vi "Settings.vi"(9 "Debug":bool, 10 "AeroQuad Flight Software Folder":path, 11 "Arduino IDE Folder":path) -> (1 "Debug Out":bool, 2 "Flight Software Path":path, 3 "IDE Path":path)   [LabVIEW 2010]
panel:
  in  "Cancel":bool
  in  "OK":bool
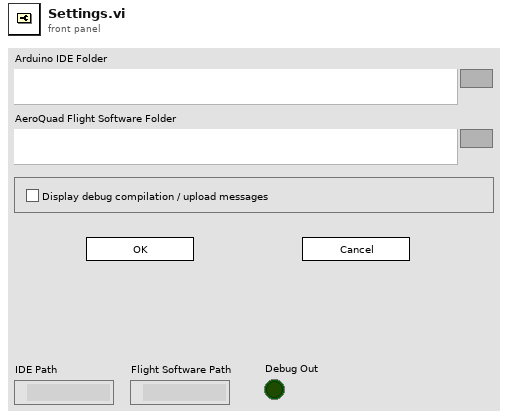
[diagram p1: front panel]
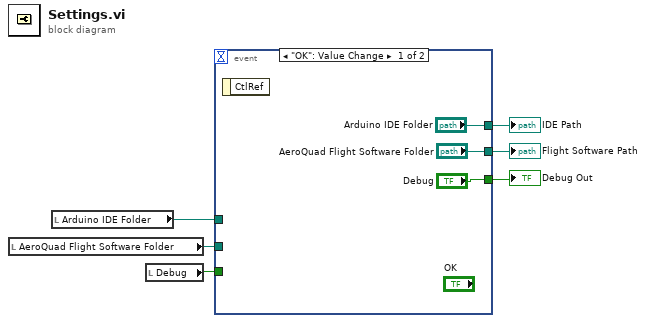
[diagram p0: block diagram]
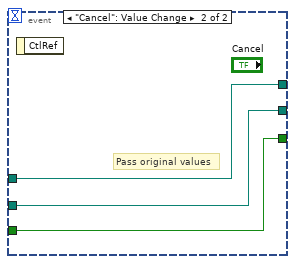
[diagram p2: hidden frame]
diagram:
  n1 = local read "AeroQuad Flight Software Folder"() -> (w2:path)
  n2 = local read "Arduino IDE Folder"() -> (w3:path)
  n3 = local read "Debug"() -> (w1:bool)
  n4 = event shown="[0] \"OK\": Value Change" {
    selector: _ -> [_ _]
    dyn-events: _ -> [_ _]
    timeout: _ -> [_ _]
    tunnel: ["Arduino IDE Folder" w12] -> w6
    tunnel: ["AeroQuad Flight Software Folder" w11] -> w5
    tunnel: ["Debug" w10] -> w4
    tunnel: w3 -> [_ w12]
    tunnel: w2 -> [_ w11]
    tunnel: w1 -> [_ w10]
    event "OK": Value Change {
      n5 = event-data() -> ()  [unwired: 1 in, 1 out]
    }
    event "Cancel": Value Change {
      # "Pass original values"
      n6 = event-data() -> ()  [unwired: 1 in, 1 out]
    }
  }
  "IDE Path" <- w6
  "Flight Software Path" <- w5
  "Debug Out" <- w4
